vi "Start Storage.vi"(8 "error in (no error)":errorcluster, 10 "Storage Key Expression":string="myhome/kitchen/temp", 11 "Zenoh in":refnum<class "Zenoh.lvclass">) -> (0 "error out":errorcluster, 3 "Zenoh out":refnum<class "Zenoh.lvclass">)   [LabVIEW 2021, in "Zenoh.lvclass"]
uses:
  Zenoh.lvclass
  Zenoh.lvclass/Zenoh.ctl
  typedef/Storage Info.ctl
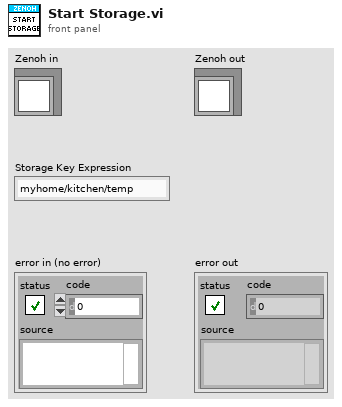
[diagram p1: front panel]
types:
  T1 = typedef "Zenoh.lvclass/Storage Info.ctl" = cluster{"Storage Handle":u64}
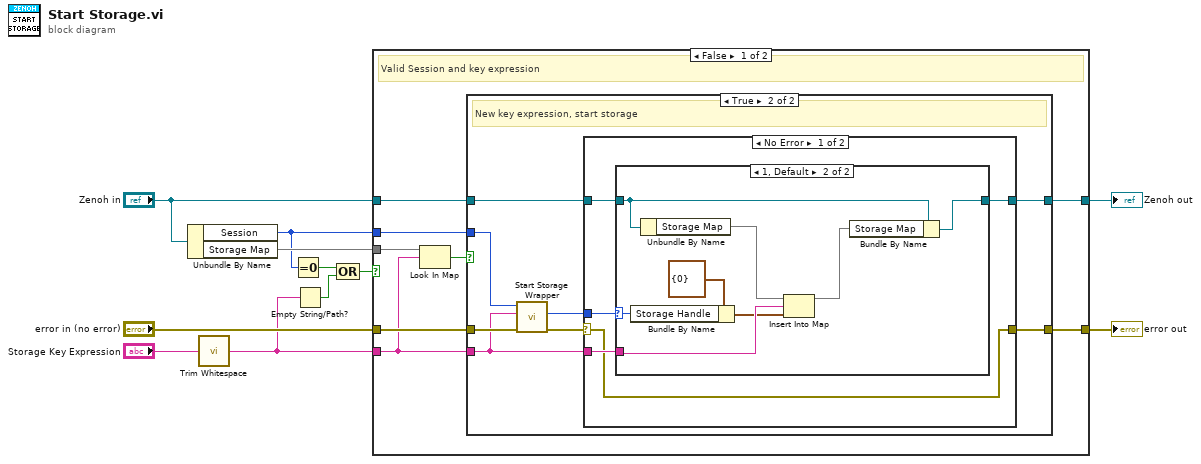
[diagram p0: block diagram]
diagram:
  n1 = Unbundle By Name("Zenoh in") -> ("Session"=w1:u64, "Storage Map"=w9:map{string, T1})
  n2 = call <vilib>:"Trim Whitespace.vi"("string"="Storage Key Expression") -> ("trimmed string"=w5:string)  [unwired: 1 in]
  n3 = Equal To 0?(x=w1) -> (x = 0?=w4:bool)
  n4 = Empty String/Path?(string/path=w5) -> (empty?=w3:bool)
  n5 = Compound Arithmetic op=OR(w4, w3) -> (w2:bool)
  n6 = case shown="False" w2 {
    tunnel: w5 -> [w16 _]
    tunnel: "error in (no error)" -> [w19 w46]
    tunnel: "Zenoh in" -> [w17 w47]
    tunnel: w9 -> [w18 _]
    tunnel: [w15 w46] -> w8
    tunnel: [w14 w47] -> w7
    tunnel: w1 -> [w12 _]
    frame False {
      # "Valid Session and key expression"
      n7 = Look In Map(map=w18, key=w16) -> (key not found?=w13:bool)  [unwired: 1 in, 1 out]
      n8 = case shown="True" w13 {
        tunnel: w19 -> [w20 w26]
        tunnel: w12 -> [_ w24]
        tunnel: w17 -> [w21 w29]
        tunnel: w16 -> [_ w25]
        tunnel: [w20 w28] -> w15
        tunnel: [w21 w27] -> w14
        frame False {
          # "Storage already created with this key expression"
        }
        frame True {
          # "New key expression, start storage"
          n9 = call "Start Storage Wrapper.vi"("error in (no error)"=w26, "Key Expression"=w25, "Session in"=w24) -> ("error out"=w23:errorcluster, "Storage Handle"=w22:u64)  [unwired: 7 in]
          n10 = case shown="No Error" w23 {
            selector: w23 -> [w30 w44]
            tunnel: w22 -> [w34 _]
            tunnel: w29 -> [w33 w45]
            tunnel: w25 -> [w32 _]
            tunnel: [w31 w45] -> w27
            tunnel: [w30 w44] -> w28
            frame No Error {
              n11 = case shown="1, Default" w34 {
                selector: w34 -> [_ w41]
                tunnel: w33 -> [w35 w39]
                tunnel: w32 -> [_ w42]
                tunnel: [w35 w37] -> w31
                frame 0 {
                }
                frame 1, Default {
                  n12 = Bundle By Name(cluster=T1 {"Storage Handle"=0} ("Storage"), "Storage Handle"=w41) -> (w40:T1)
                  n13 = Unbundle By Name(w39) -> ("Storage Map"=w43:map{string, T1})
                  n14 = Insert Into Map(map in=w43, key=w42, value=w40) -> (map out=w38:map{string, T1})  [unwired: 2 out]
                  n15 = Bundle By Name(cluster=w39, "Storage Map"=w38) -> (w37:refnum<class "Zenoh.lvclass">)
                }
              }
            }
            frame Error {
            }
          }
        }
      }
    }
    frame True {
      # "Invalid session or key expression"
    }
  }
  "error out" <- w8
  "Zenoh out" <- w7
